vi "IntR.vi"(2 "xpunkt(t)":dbl format="%.2f", 3 "x0":dbl format="%.2f") -> (0 "x(t)":dbl format="%.2f")   [LabVIEW 2009]
uses:
  Vibe/Delta_t.vi
panel:
  in  "Initialisieren (False)":bool
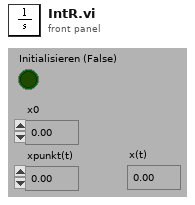
[diagram p1: front panel]
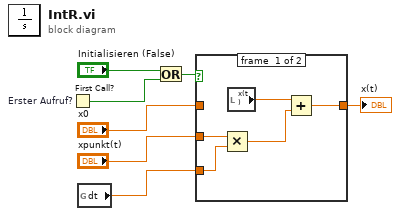
[diagram p0: block diagram]
diagram:
  n1 = First Call? "Erster Aufruf?"() -> (First Call?: T/F=w4:bool)
  n2 = global read "Delta_t.vi" "dt"() -> (w3:dbl)
  n3 = Or(x="Initialisieren (False)", y=w4) -> (x .or. y?=w2:bool)
  n4 = case shown="True" w2 {
    tunnel: "x0" -> [_ w13]
    tunnel: "xpunkt(t)" -> [w12 _]
    tunnel: w3 -> [w9 _]
    tunnel: [w8 w13] -> w1
    frame #0 {
      n5 = Multiply(x=w12, y=w9) -> (x*y=w10:dbl)
      n6 = local read "x(t)"() -> (w11:dbl)
      n7 = Add(x=w11, y=w10) -> (x+y=w8:dbl)
    }
    frame #1 {
    }
  }
  "x(t)" <- w1
